vi "Port to Read.vi"(8 "error in (no error)":errorcluster, 10 "Port to Read":dbl, 11 "Simulado in":refnum<class "Simulado.lvclass">) -> (0 "error out":errorcluster, 3 "Simulado out":refnum<class "Simulado.lvclass">)   [LabVIEW 2020, in "Simulado.lvclass"]
doc: "genera un comando para preguntar por el puerto que se quiere leer"
uses:
  Simulado.lvclass
  Simulado.lvclass/Simulado.ctl
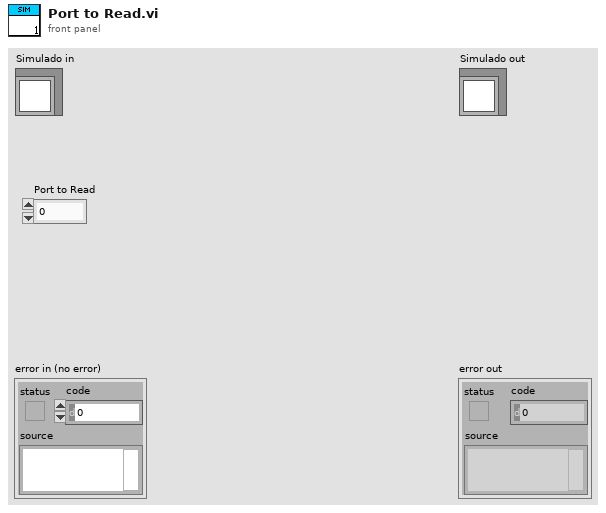
[diagram p1: front panel]
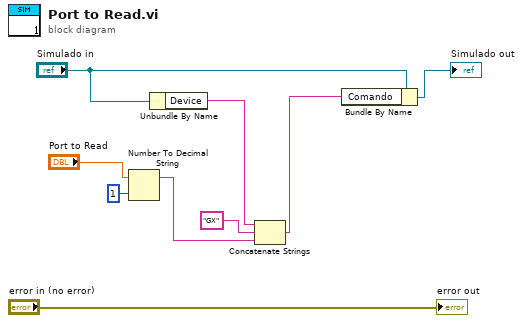
[diagram p0: block diagram]
diagram:
  n1 = Number To Decimal String(number="Port to Read", width (-)=i16 1) -> (decimal integer string=w4:string)
  n2 = Unbundle By Name("Simulado in") -> ("Device"=w6:string)
  n3 = Concatenate Strings(w6, "GX" ("string"), w4) -> (w5:string)
  n4 = Bundle By Name(cluster="Simulado in", "Comando"=w5) -> (→"Simulado out":refnum<class "Simulado.lvclass">)
  "error out" <- "error in (no error)"
